vi "Register for Laser Events.vi"(8 "error in (no error)":errorcluster, 11 "Get Laser Status in":refnum<class "Get Laser Status.lvclass">) -> (0 "error out":errorcluster, 1 "Laser Process State":refnum<event-registration>, 2 "Laser State":refnum<event-registration>, 3 "Get Laser Status out":refnum<class "Get Laser Status.lvclass">)   [LabVIEW 2022 SP3, in "Get Laser Status.lvclass"]
uses:
  Get Laser Status.lvclass
  Laser State Data/Laser State.ctl
  Laser State Data/Laser State Data.lvclass
  Laser State Data/Events.ctl
  XY Stage/Process Actor/Process Framework/Process State Data/Events.ctl
  XY Stage/Process Actor/Process Framework/Process State Data/Process State Data.lvclass
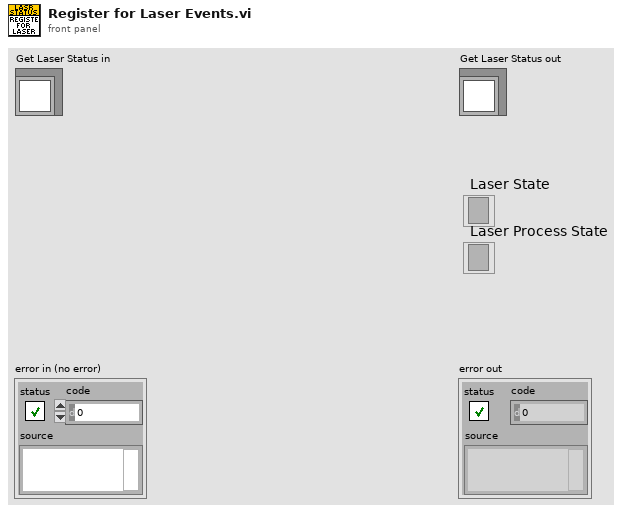
[diagram p1: front panel]
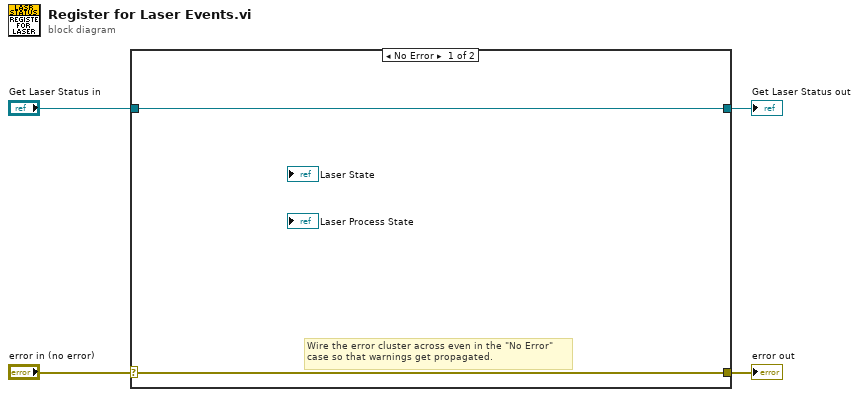
[diagram p0: block diagram]
diagram:
  n1 = case shown="No Error" "error in (no error)" {
    selector: "error in (no error)" -> [w5 w8]
    tunnel: [w5 w8] -> w3
    tunnel: [w6 w7] -> w1
    tunnel: "Get Laser Status in" -> [w6 w7]
    frame No Error {
      # "Wire the error cluster across even in the \"No Error\"\ncase so that warnings get propagated."
    }
    frame Error {
    }
  }
  "error out" <- w3
  "Get Laser Status out" <- w1
